vi "DigitalIORead.vi"(3 "error in":errorcluster, 4 "Component":T1, 5 "node":string) -> (0 "error out":errorcluster, 1 "Digital IO State":cluster{"state":i8, "is input only":bool})   [LabVIEW 2010]
uses:
  ROS/Code/SubVIs/_ROSDirection.ctl
  ROS/Code/Console/Servers/ServerSubs/TopicDef.ctl
  ROS/Code/SubVIs/DigitalIOComponents.ctl
panel:
  out "Reply":string
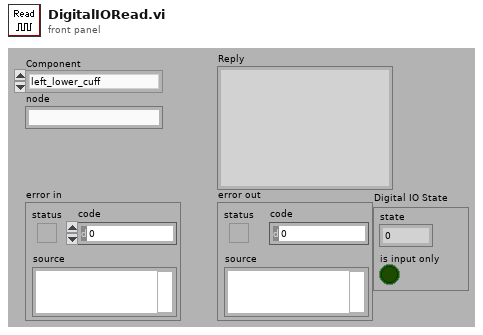
[diagram p1: front panel]
types:
  T1 = typedef "DigitalIOComponents.ctl" = enum16{"left_lower_cuff", "right_lower_cuff", "left_lower_button", "right_lower_button", "left_upper_button", "right_upper_button", "left_shoulder_button", "right_shoulder_button"}
  T2 = typedef "TopicDef.ctl" = cluster{"Topic":string, "Type":string, "Action":T3, "Update (ms)":u16, "write queue":u16}
  T3 = typedef "_ROSDirection.ctl" = enum16{"Node", "Publisher", "Subscriber", "Service Client"}
  T4 = typedef "_ROSControl.ctl" = cluster{"topic port":u16, "Node":string, "topic":string, "type":string, "node port":u32, "error ":errorcluster, "Direction":T3, "APIs":string[], "Update (ms)":u16, "write queue":u16}
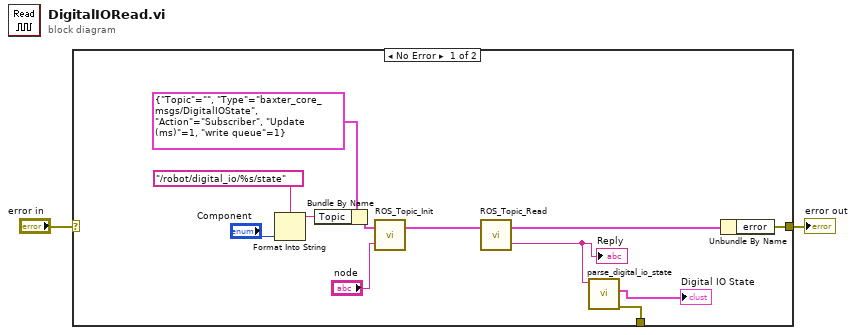
[diagram p0: block diagram]
diagram:
  n1 = case shown="No Error" "error in" {
    selector: "error in" -> [_ w15]
    tunnel: [w14 w15] -> w2
    tunnel: [w8 _] -> _
    frame No Error {
      n2 = Format Into String(format string="/robot/digital_io/%s/state" ("topic"), "Component") -> (resulting string=w5:string)  [unwired: 2 in, 1 out]
      n3 = Bundle By Name(cluster=T2 {"Topic"="", "Type"="baxter_core_msgs/DigitalIOState", "Action"=enum."Subscriber", "Update (ms)"=1, "write queue"=1} ("Definitions"), "Topic"=w5) -> (w4:T2)
      n4 = call "ROS_Topic_Init.vi"("node"="node", "Definitions"=w4) -> ("ROS out"=w12:T4)  [unwired: 1 in]
      n5 = call "ROS_Topic_Read.vi"("ROS in"=w12) -> ("Reply"=w10:string, "ROS out"=w11:T4)  [unwired: 1 in]
      "Reply" <- w10
      n6 = call "parse_digital_io_state.vi"("msg in"=w10) -> ("error out"=w8:errorcluster, "Digital IO State"=→"Digital IO State":cluster{"state":i8, "is input only":bool})  [unwired: 4 in, 1 out]
      n7 = Unbundle By Name(w11) -> ("error"=w14:errorcluster)
    }
    frame Error {
    }
  }
  "error out" <- w2
